vi "DefaultToIni.vi"(8 "error in (no error)":errorcluster, 11 "SamplerPluginsBase in":refnum<class "SamplerPluginsBase.lvclass">) -> (0 "error out":errorcluster, 3 "SamplerPluginsBase out":refnum<class "SamplerPluginsBase.lvclass">)   [LabVIEW 2014, in "SamplerPlugins.lvlib" / "SamplerPluginsBase.lvclass"]
uses:
  SamplerPluginsBase.lvclass
  TypeDefs/DefaultINIParams.ctl
  <userlib>/NIST/BaseClasses/BasePlugin_class/BasePlugin.lvclass/BasePlugin.ctl
  <userlib>/NIST/BaseClasses/BasePlugin_class/Accessors/Read PluginIniFilePath.vi
  <vilib>/Utility/config.llb/NI_LVConfig.lvlib
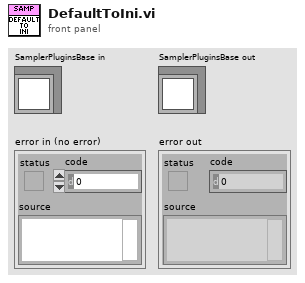
[diagram p1: front panel]
types:
  T1 = typedef "SamplerPlugins.lvlib/SamplerPluginsBase.lvclass/DefaultINIParams.ctl" = cluster{"Handle":string, "eFunction":u16, "dRange":dbl, "dResolution":dbl, "eTriggerSource":u16, "dTriggerDelay":dbl, "iMaxTimeMilliseconds":i32, "eMeasCompleteDest":u16, "iTriggerCount":i32, "iSampleCount":i32, "eSampleClock":u16, "dSampleInterval":dbl, "iMaxTimeMillisecondsMultiPoint":i32, "iArraySize":i32, "dMinFreq":dbl, "dMaxFreq":dbl, "dFrequencyVoltageRange":dbl, "eEdge":u16, "sSource":string, "eEdgeSample":u16, "sSourceSample":string}
  T2 = typedef "SamplerPlugins.lvlib/SamplerPluginsBase.lvclass/ConfigMultiPointParams.ctl" = cluster{"iTriggerCount":i32, "iSampleCount":i32, "eSampleClock":u16, "dSampleInterval":dbl}
  T3 = typedef "SamplerPlugins.lvlib/SamplerPluginsBase.lvclass/MultiPointParams.ctl" = cluster{"iMaxTimeMilliseconds":i32, "iArraySize":i32}
  T4 = typedef "SamplerPlugins.lvlib/SamplerPluginsBase.lvclass/ConfigACBandwidthParams.ctl" = cluster{"dMinFreq":dbl, "dMaxFreq":dbl}
  T5 = typedef "SamplerPlugins.lvlib/SamplerPluginsBase.lvclass/TriggerParams.ctl" = cluster{"eEdge":u16, "sSource":string}
  T6 = typedef "NI_LVConfig.lvlib/Config Data RefNum.ctl" = refnum<k1>
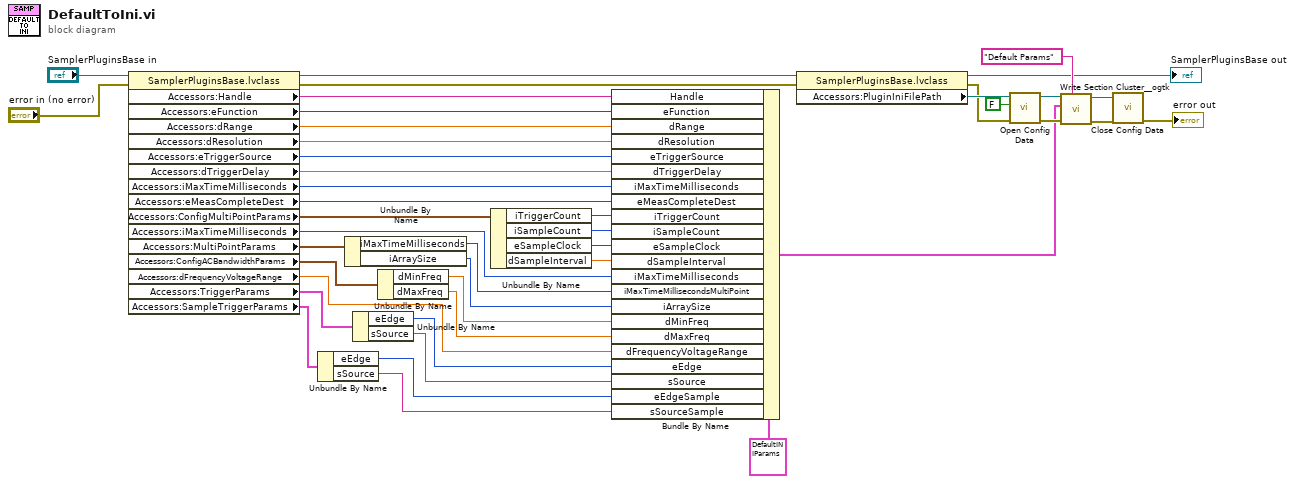
[diagram p0: block diagram]
diagram:
  n1 = property class="SamplerPluginsBase.lvclass"(reference="SamplerPluginsBase in", error in="error in (no error)") -> (reference out=w13:refnum<class "SamplerPluginsBase.lvclass">, error out=w12:errorcluster, "Accessors:Handle"=w41:string, "Accessors:eFunction"=w40:u16, "Accessors:dRange"=w39:dbl, "Accessors:dResolution"=w38:dbl, "Accessors:eTriggerSource"=w37:u16, "Accessors:dTriggerDelay"=w36:dbl, "Accessors:iMaxTimeMilliseconds"=w35:i32, "Accessors:eMeasCompleteDest"=w34:u16, "Accessors:ConfigMultiPointParams"=w33:T2, "Accessors:iMaxTimeMilliseconds"=w28:i32, "Accessors:MultiPointParams"=w25:T3, "Accessors:ConfigACBandwidthParams"=w24:T4, "Accessors:dFrequencyVoltageRange"=w21:dbl, "Accessors:TriggerParams"=w20:T5, "Accessors:SampleTriggerParams"=w17:T5)
  n2 = Unbundle By Name(w17) -> ("eEdge"=w16:u16, "sSource"=w15:string)
  n3 = Unbundle By Name(w25) -> ("iMaxTimeMilliseconds"=w27:i32, "iArraySize"=w26:i32)
  n4 = Unbundle By Name(w20) -> ("eEdge"=w19:u16, "sSource"=w18:string)
  n5 = Unbundle By Name(w24) -> ("dMinFreq"=w23:dbl, "dMaxFreq"=w22:dbl)
  n6 = Unbundle By Name(w33) -> ("iTriggerCount"=w32:i32, "iSampleCount"=w31:i32, "eSampleClock"=w30:u16, "dSampleInterval"=w29:dbl)
  n7 = Bundle By Name(cluster=T1 {"Handle"="", "eFunction"=0, "dRange"=0.0, "dResolution"=0.0, "eTriggerSource"=0, "dTriggerDelay"=0.0, "iMaxTimeMilliseconds"=0, "eMeasCompleteDest"=0, "iTriggerCount"=0, "iSampleCount"=0, "eSampleClock"=0, "dSampleInterval"=0.0, "iMaxTimeMillisecondsMultiPoint"=0, "iArraySize"=0, "dMinFreq"=0.0, "dMaxFreq"=0.0, "dFrequencyVoltageRange"=0.0, "eEdge"=10280, "sSource"="", "eEdgeSample"=10280, "sSourceSample"=""} ("DefaultINIParams"), "Handle"=w41, "eFunction"=w40, "dRange"=w39, "dResolution"=w38, "eTriggerSource"=w37, "dTriggerDelay"=w36, "iMaxTimeMilliseconds"=w35, "eMeasCompleteDest"=w34, "iTriggerCount"=w32, "iSampleCount"=w31, "eSampleClock"=w30, "dSampleInterval"=w29, "iMaxTimeMilliseconds"=w28, "iMaxTimeMillisecondsMultiPoint"=w27, "iArraySize"=w26, "dMinFreq"=w23, "dMaxFreq"=w22, "dFrequencyVoltageRange"=w21, "eEdge"=w19, "sSource"=w18, "eEdgeSample"=w16, "sSourceSample"=w15) -> (w6:T1)
  n8 = property class="SamplerPluginsBase.lvclass"(reference=w13, error in=w12) -> (reference out=→"SamplerPluginsBase out":refnum<class "SamplerPluginsBase.lvclass">, error out=w9:errorcluster, "Accessors:PluginIniFilePath"=w11:path)
  n9 = call <vilib>:"Open Config Data.vi"("error in (no error)"=w9, "create file if necessary (T)"=FALSE, "configuration file path"=w11) -> ("error out"=w8:errorcluster, "refnum"=w7:T6)  [unwired: 6 in, 1 out]
  n10 = call <userlib>:"Write Section Cluster__ogtk.vi"("section (optional)"="Default Params", "error in (no error)"=w8, "Section Formatted Cluster"=w6, "refnum"=w7) -> ("error out"=w4:errorcluster, "dup refnum"=w3:T6)  [unwired: 6 in]
  n11 = call <vilib>:"Close Config Data.vi"("error in (no error)"=w4, "refnum"=w3) -> ("error out"=→"error out":errorcluster)  [unwired: 8 in, 1 out]
